vi "GET_Initial_SubCondition_representation.vi"(2 "error in (no error)":errorcluster, 3 "Input parameters cluster":T9 {"Array of conditions in"."Specifier(s)"."Validity criteria(s)"."Validity value" min=0.0 step=0.1 format="%.2g"; "Array of conditions in"."Specifier(s)"."Value" step=1.0 format="%#.2g"; "Calibration parameters"."True frame time, s" format="%.10g"; "Calibration parameters"."Disp. calibration info"."Speed, µl per ms" format="%.3g"; "Calibration parameters"."True FPS" format="%.10g"; "Calibration parameters"."Timing calibration sw/hw" format="%.10g"}) -> (0 "error out":errorcluster, 1 "Output parameters cluster":T1 {"SubCondition"."Specifier(s)"."Validity criteria(s)"."Validity value" min=0.0 step=0.1 format="%.2g"; "SubCondition"."Specifier(s)"."Value" step=1.0 format="%#.2g"})   [LabVIEW 2018, in "Tracker.lvlib"]
uses:
  Tracker.lvlib
  Controls/CTL_Conditions_build_parameters_in.ctl
  Controls/CTL_Conditions_Array.ctl
  Controls/CTL_Conditions_Cluster.ctl
  Controls/CTL_Condition_type.ctl
  Controls/CTL_Comparison_type.ctl
  Controls/CTL_Validity_check_criteria.ctl
  Controls/CTL_Response_info.ctl
  Controls/CTL_Condition_response_type.ctl
  Controls/CTL_Reponse_port_info.ctl
  Controls/CTL_Calibration_parameters.ctl
  Controls/CTL_Dispenser_calibration_info.ctl
  Controls/CTL_Conditions_build_parameters_out.ctl
  Common_Resources.lvlib
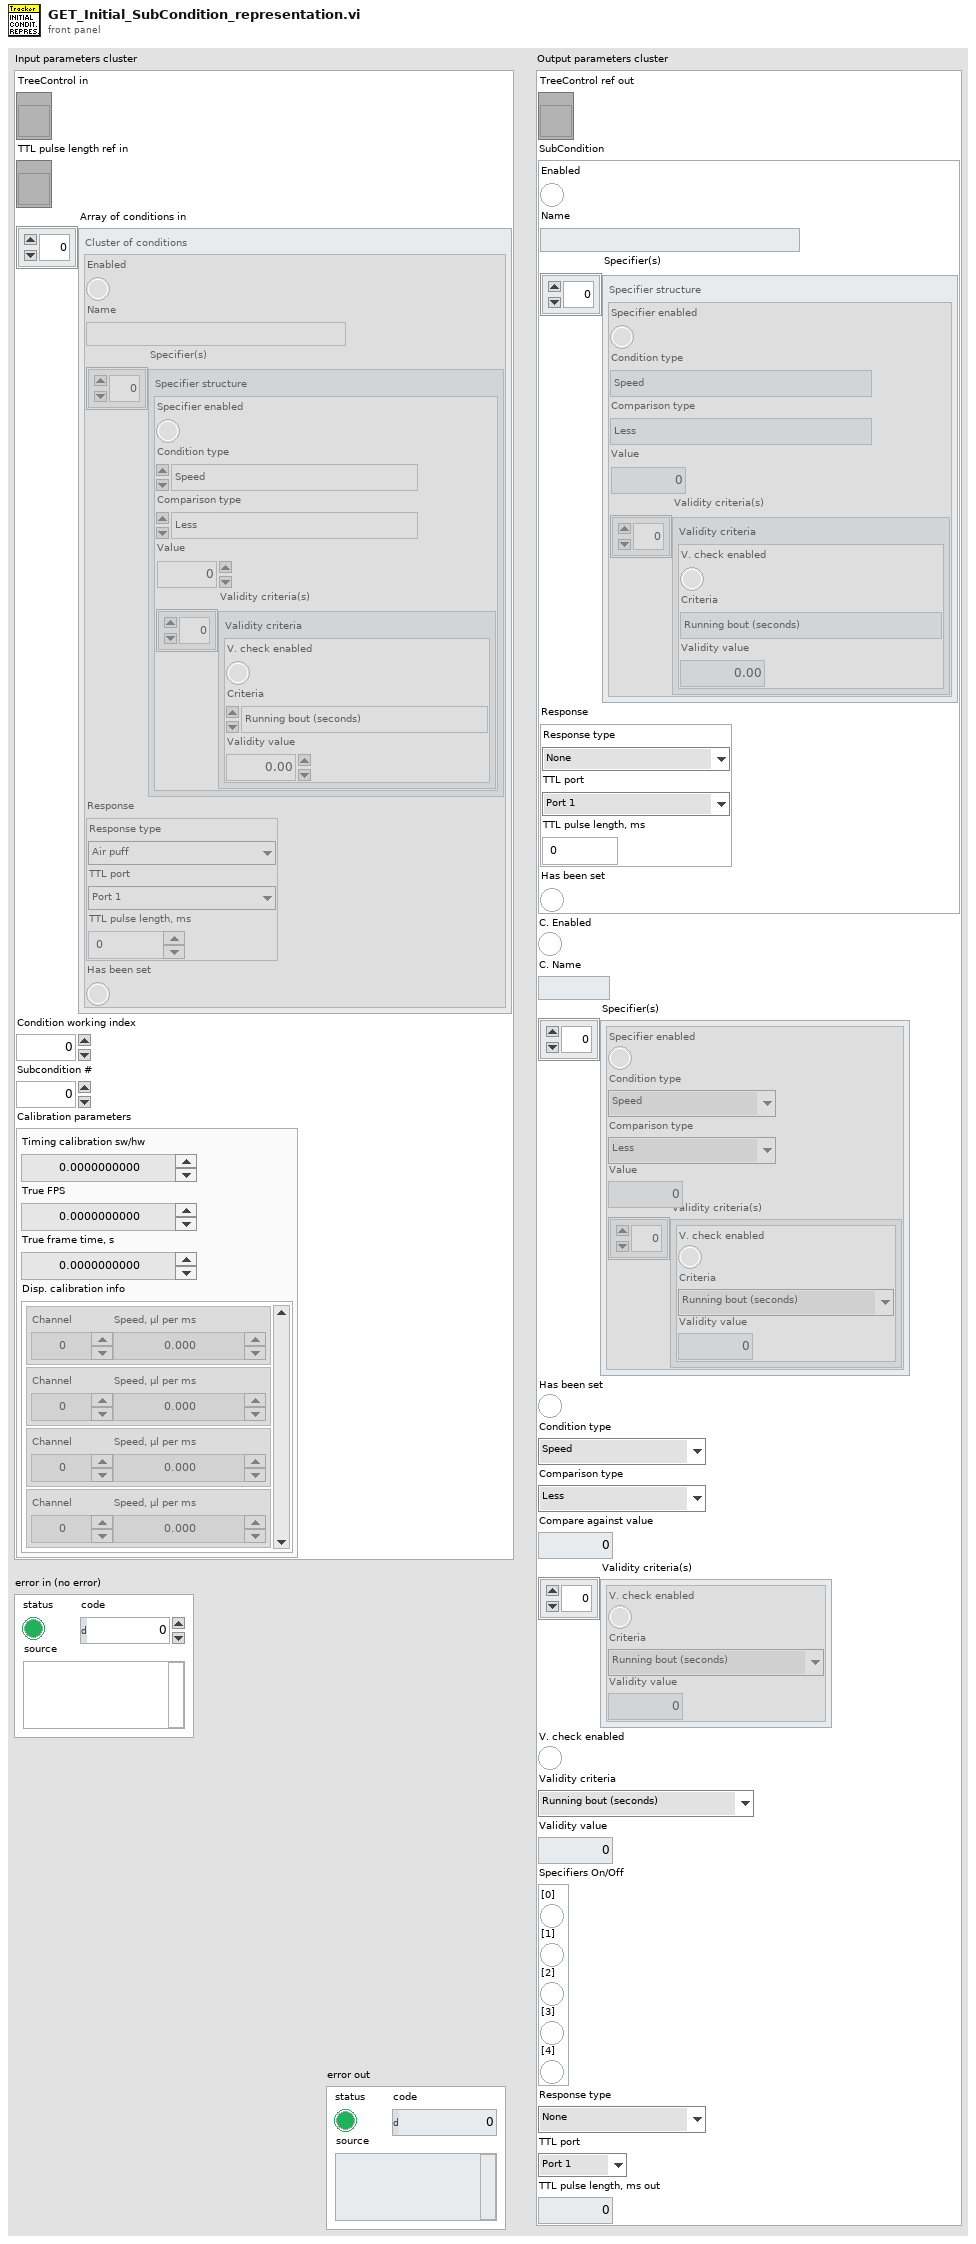
[diagram p1: front panel]
types:
  T1 = typedef "Common_Resources.lvlib/CTL_Conditions_build_parameters_out.ctl" = cluster{"TreeControl ref out":refnum<vi>, "SubCondition":T2, "C. Enabled":bool, "C. Name":string, "Specifier(s)":cluster{"Specifier enabled":bool, "Condition type":T3, "Comparison type":T4, "Value":dbl, "Validity criteria(s)":cluster{"V. check enabled":bool, "Criteria":T5, "Validity value":dbl}[]}[], "Has been set":bool, "Condition type":T3, "Comparison type":T4, "Compare against value":dbl, "Validity criteria(s)":cluster{"V. check enabled":bool, "Criteria":T5, "Validity value":dbl}[], "V. check enabled":bool, "Validity criteria":T5, "Validity value":dbl, "Specifiers On/Off":cluster{"[0]":bool, "[1]":bool, "[2]":bool, "[3]":bool, "[4]":bool}, "Response type":T7, "TTL port":T8, "TTL pulse length, ms out":dbl}
  T2 = typedef "Common_Resources.lvlib/CTL_Conditions_Cluster.ctl" = cluster{"Enabled":bool, "Name":string, "Specifier(s)":cluster{"Specifier enabled":bool, "Condition type":T3, "Comparison type":T4, "Value":dbl, "Validity criteria(s)":cluster{"V. check enabled":bool, "Criteria":T5, "Validity value":dbl}[]}[], "Response":T6, "Has been set":bool}
  T3 = typedef "Common_Resources.lvlib/CTL_Condition_type.ctl" = enum16{"Speed", "Zone", "Angle to wall"}
  T4 = typedef "Common_Resources.lvlib/CTL_Comparison_type.ctl" = enum16{"Less", "Less or Equal", "Equal", "Greater or Equal", "Greater", "Not Equal"}
  T5 = typedef "Common_Resources.lvlib/CTL_Validity_check_criteria.ctl" = enum16{"Running bout (seconds)", "Running bout (meters)"}
  T6 = typedef "Common_Resources.lvlib/CTL_Response_info.ctl" = cluster{"Response type":T7, "TTL port":T8, "TTL pulse length, ms":dbl}
  T7 = typedef "Common_Resources.lvlib/CTL_Condition_response_type.ctl" = enum16{"None", "Air puff", "Liquid reward"}
  T8 = typedef "Common_Resources.lvlib/CTL_Reponse_port_info.ctl" = enum16{"Port 1", "Port 2", "Port 3", "Port 4"}
  T9 = typedef "Common_Resources.lvlib/CTL_Conditions_build_parameters_in.ctl" = cluster{"TreeControl in":refnum<vi>, "TTL pulse length ref in":refnum<vi>, "Array of conditions in":T10, "Condition working index":i32, "Subcondition #":i32, "Calibration parameters":T11}
  T10 = typedef "Common_Resources.lvlib/CTL_Conditions_Array.ctl" = T2[]
  T11 = typedef "Common_Resources.lvlib/CTL_Calibration_parameters.ctl" = cluster{"Timing calibration sw/hw":dbl, "True FPS":dbl, "True frame time, s":dbl, "Disp. calibration info":T12}
  T12 = typedef "Common_Resources.lvlib/CTL_Dispenser_calibration_info.ctl" = cluster{"Channel":u8, "Speed, µl per ms":dbl}[]
  T13 = cluster{"Specifier enabled":bool, "Condition type":T3, "Comparison type":T4, "Value":dbl, "Validity criteria(s)":cluster{"V. check enabled":bool, "Criteria":T5, "Validity value":dbl}[]}[]
  T14 = cluster{"Specifier enabled":bool, "Condition type":T3, "Comparison type":T4, "Value":dbl, "Validity criteria(s)":cluster{"V. check enabled":bool, "Criteria":T5, "Validity value":dbl}[]}
  T15 = cluster{"V. check enabled":bool, "Criteria":T5, "Validity value":dbl}[]
  T16 = cluster{"V. check enabled":bool, "Criteria":T5, "Validity value":dbl}
  T17 = cluster{"[0]":bool, "[1]":bool, "[2]":bool, "[3]":bool, "[4]":bool}
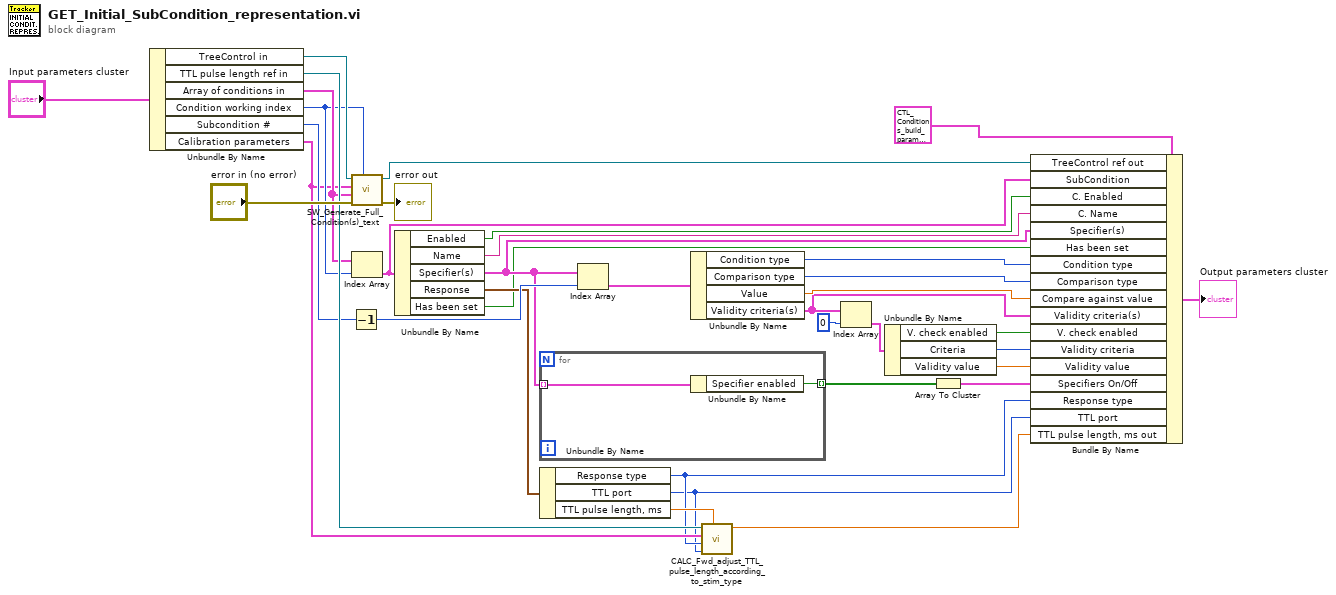
[diagram p0: block diagram]
diagram:
  n1 = Unbundle By Name("Input parameters cluster") -> ("TreeControl in"=w25:refnum<vi>, "TTL pulse length ref in"=w26:refnum<vi>, "Array of conditions in"=w24:T10, "Condition working index"=w23:i32, "Subcondition #"=w22:i32, "Calibration parameters"=w21:T11)
  n2 = Decrement(x=w22) -> (x-1=w33:i32)
  n3 = call "SW_Generate_Full_Condition(s)_text.vi"("Array index to show"=w23, "error in (no error)"="error in (no error)", "Array of conditions in"=w24, "Calibration parameters"=w21, "TreeControl ref in"=w25) -> ("error out"=→"error out":errorcluster, "TreeControl ref out"=w19:refnum<vi>)  [unwired: 5 in]
  n4 = Index Array(array=w24, index=w23) -> (element=w18:T2)
  n5 = Unbundle By Name(w18) -> ("Enabled"=w14:bool, "Name"=w13:string, "Specifier(s)"=w8:T13, "Response"=w20:T6, "Has been set"=w4:bool)
  n6 = for {
    tunnel: w8 -> [w37] mode=indexing
    tunnel: [w36] -> w32 mode=indexing
    n7 = Unbundle By Name(w37) -> ("Specifier enabled"=w36:bool)
  }
  n8 = Unbundle By Name(w20) -> ("Response type"=w6:T7, "TTL port"=w1:T8, "TTL pulse length, ms"=w31:dbl)
  n9 = Index Array(array=w8, index=w33) -> (element=w28:T14)
  n10 = Unbundle By Name(w28) -> ("Condition type"=w17:T3, "Comparison type"=w16:T4, "Value"=w15:dbl, "Validity criteria(s)"=w12:T15)
  n11 = call "CALC_Fwd_adjust_TTL_pulse_length_according_to_stim_type.vi"("TTL pulse length, ms in"=w31, "TTL port"=w1, "Response type"=w6, "Calibration parameters"=w21, "TTL pulse length ref in"=w26) -> ("TTL pulse length, ms out"=w5:dbl)  [unwired: 6 in]
  n12 = Index Array(array=w12, index=0) -> (element=w30:T16)
  n13 = Unbundle By Name(w30) -> ("V. check enabled"=w11:bool, "Criteria"=w10:T5, "Validity value"=w9:dbl)
  n14 = Array To Cluster(array=w32) -> (cluster=w7:T17)
  n15 = Bundle By Name(cluster=T1 {"TreeControl ref out"=refnum, "SubCondition"={"Enabled"=FALSE, "Name"="", "Specifier(s)"=[], "Response"={"Response type"=enum."None", "TTL port"=enum."Port 1", "TTL pulse length, ms"=0.0}, "Has been set"=FALSE}, "C. Enabled"=FALSE, "C. Name"="", "Specifier(s)"=[], "Has been set"=FALSE, "Condition type"=enum."Speed", "Comparison type"=enum."Less", "Compare against value"=0.0, "Validity criteria(s)"=[], "V. check enabled"=FALSE, "Validity criteria"=enum."Running bout (seconds)", "Validity value"=0.0, "Specifiers On/Off"={"[0]"=FALSE, "[1]"=FALSE, "[2]"=FALSE, "[3]"=FALSE, "[4]"=FALSE}, "Response type"=enum."None", "TTL port"=enum."Port 1", "TTL pulse length, ms out"=0.0} ("Output parameters cluster"), "TreeControl ref out"=w19, "SubCondition"=w18, "C. Enabled"=w14, "C. Name"=w13, "Specifier(s)"=w8, "Has been set"=w4, "Condition type"=w17, "Comparison type"=w16, "Compare against value"=w15, "Validity criteria(s)"=w12, "V. check enabled"=w11, "Validity criteria"=w10, "Validity value"=w9, "Specifiers On/Off"=w7, "Response type"=w6, "TTL port"=w1, "TTL pulse length, ms out"=w5) -> (→"Output parameters cluster":T1)
